vi "MCCMSG Set Pipette Offset.vi"(8 "error in (no error)":errorcluster, 9 "pnError":i32, 10 "dPipetteOffset":dbl, 11 "hMCCmsg":i32) -> (0 "error out":errorcluster, 1 "pnError out":i32, 3 "function return":i32)   [LabVIEW 2012, in "MultiClamp 700B Controls.lvlib" / "AxMultiClampMsg.lvlib"]
doc: "AXMCCMSG BOOL WINAPI MCCMSG_SetPipetteOffset(HMCCMSG hMCCmsg, double dPipetteOffset, int *pnError);"
uses:
  AxMultiClampMsg.lvlib
  AxMultiClampMsg.dll
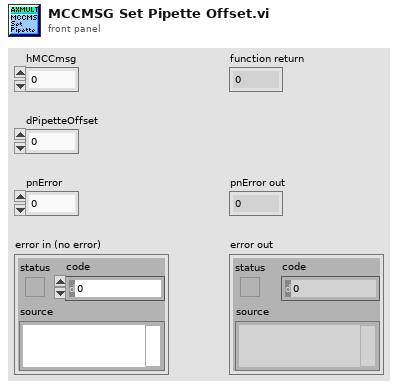
[diagram p1: front panel]
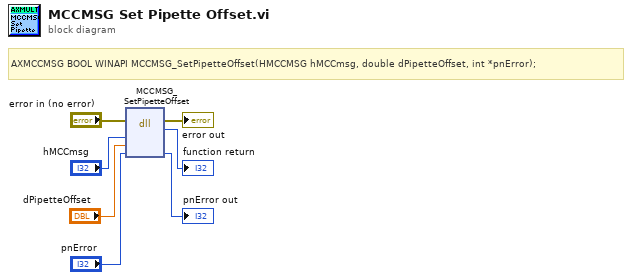
[diagram p0: block diagram]
diagram:
  # "AXMCCMSG BOOL WINAPI MCCMSG_SetPipetteOffset(HMCCMSG hMCCmsg, double dPipetteOffset, int *pnError);"
  n1 = dll-call lib="C:/Users/Southampton/Desktop/Rita/Multiclamp 700B VIs/AxMultiClampMsg/AxMultiClampMsg.*" fn="MCCMSG_SetPipetteOffset"(error in="error in (no error)", "hMCCmsg"="hMCCmsg", "dPipetteOffset"="dPipetteOffset", "pnError"="pnError") -> (error out=→"error out":errorcluster, →"function return":i32, "pnError"=→"pnError out":i32)  [unwired: 4 in, 1 out]
